vi "Initialize RF Sessions.vi"(0 "RF Subsystem Session Provider in":refnum<class "RF Subsystem Session Provider.lvclass">, 5 "TSM Context":T1, 11 "error in":errorcluster) -> (4 "RF Subsystem Session Provider out":refnum<class "RF Subsystem Session Provider.lvclass">, 15 "error out":errorcluster)   [LabVIEW 2023, in "RFFixtureCharact.RMM.lvlib" / "RF Subsystem Session Provider.lvclass"]
uses:
  RF Subsystem Session Provider.lvclass
  <vilib>/NI_TestStand_SemiconductorModule/NI_TestStand_Semiconductor_Module.lvlibp/PinMap/General/SemiconductorModuleContext.ctl
  Common/RF Subsystem Session Provider/Utilities/Global Data Id Prefix.vi
  <vilib>/NI_TestStand_SemiconductorModule/NI_TestStand_Semiconductor_Module.lvlibp/PinMap/Site and Global Data/SetGlobalData.vi
  RF Subsystem Session Provider.lvclass/RF Subsystem Session Provider.ctl
  <vilib>/NI_TestStand_SemiconductorModule/NI_TestStand_Semiconductor_Module.lvlibp
  Common/RFCalAndFixtureCharact.Common.lvlib
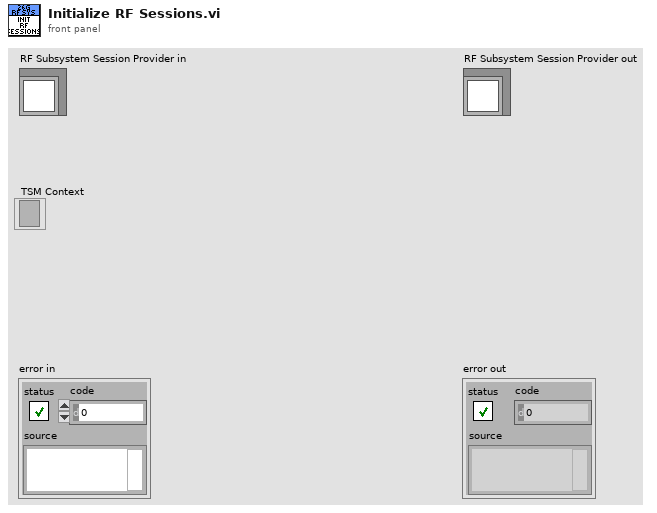
[diagram p1: front panel]
types:
  T1 = typedef "NI_TestStand_Semiconductor_Module.lvlibp/SemiconductorModuleContext.ctl" = refnum<k7>
  T2 = enum16{"OnboardClock", "RefIn", "PXI_Clk", "ClkIn", "RefIn2", "PXI_ClkMaster"}
  T3 = typedef "NI_TestStand_Semiconductor_Module.lvlibp/ModelBasedInstrumentInstanceData.ctl" = cluster{"Instrument Name":string, "Instrument Model":string}
  T4 = typedef "NI_TestStand_Semiconductor_Module.lvlibp/ModelBasedResourcePropertyList.ctl" = cluster{"Instrument Resource":string, "Properties":T5[]}
  T5 = typedef "NI_TestStand_Semiconductor_Module.lvlibp/ModelBasedInstrumentProperty.ctl" = cluster{"Property Name":string, "Property Value":string}
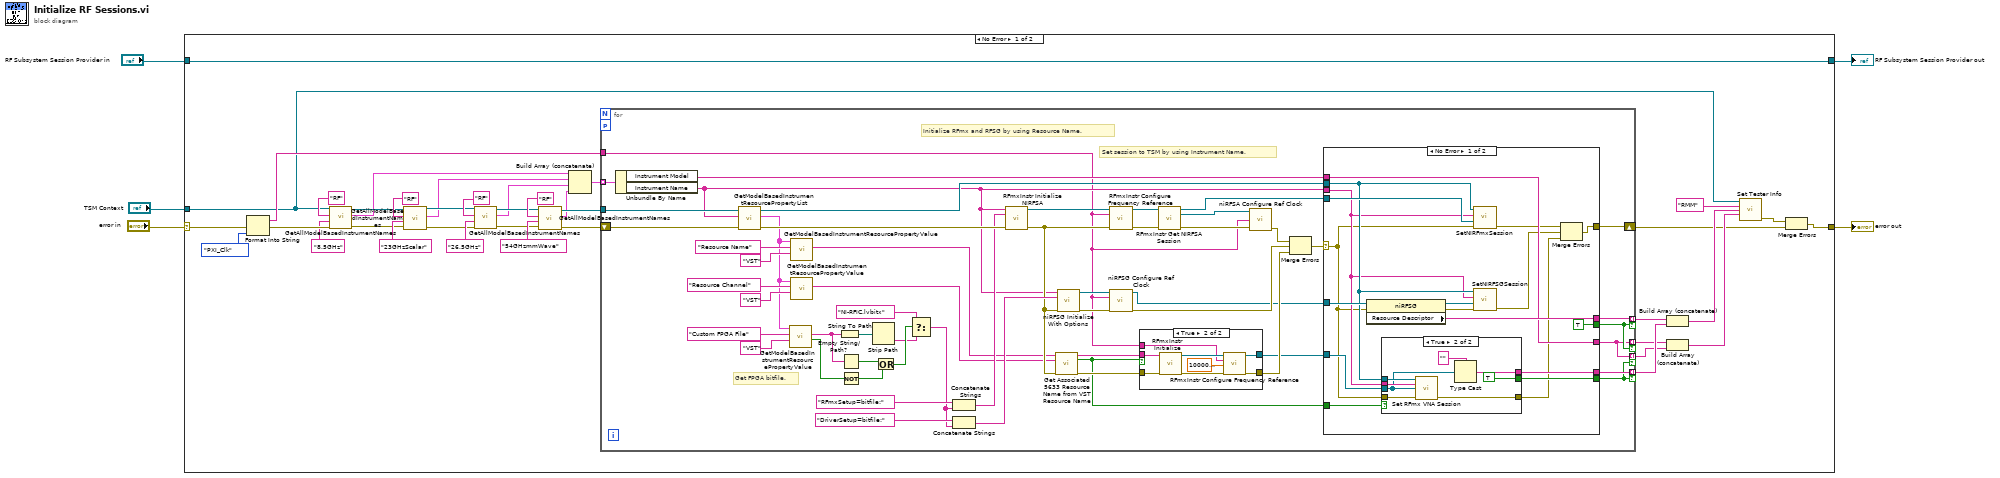
[diagram p0: block diagram]
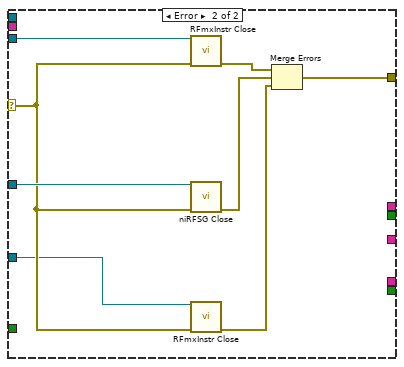
[diagram p3: hidden frame]
diagram:
  n1 = case shown="No Error" "error in" {
    selector: "error in" -> [w39 w142]
    tunnel: [w7 w142] -> w3
    tunnel: "TSM Context" -> [w17 _]
    tunnel: "RF Subsystem Session Provider in" -> [w40 w141]
    tunnel: [w40 w141] -> w1
    frame No Error {
      n2 = Format Into String(error in=w39, T2."PXI_Clk" ("Reference Clock Source In")) -> (resulting string=w37:string, error out=w20:errorcluster)  [unwired: 2 in]
      n3 = call <vilib>:"GetAllModelBasedInstrumentNames.vi"("error in (no error)"=w20, "Subcategory"="8.5GHz", "Category"="RF", "Semiconductor Module Context"=w17) -> ("error out"=w21:errorcluster, "Model-Based Instruments"=w16:T3[], "Semiconductor Module Context Out"=w18:T1)  [unwired: 5 in]
      n4 = call <vilib>:"GetAllModelBasedInstrumentNames.vi"("error in (no error)"=w21, "Subcategory"="23GHzScalar", "Category"="RF", "Semiconductor Module Context"=w18) -> ("error out"=w28:errorcluster, "Model-Based Instruments"=w24:T3[], "Semiconductor Module Context Out"=w25:T1)  [unwired: 5 in]
      n5 = call <vilib>:"GetAllModelBasedInstrumentNames.vi"("error in (no error)"=w28, "Subcategory"="26.5GHz", "Category"="RF", "Semiconductor Module Context"=w25) -> ("error out"=w27:errorcluster, "Model-Based Instruments"=w23:T3[], "Semiconductor Module Context Out"=w26:T1)  [unwired: 5 in]
      n6 = call <vilib>:"GetAllModelBasedInstrumentNames.vi"("error in (no error)"=w27, "Subcategory"="54GHzmmWave", "Category"="RF", "Semiconductor Module Context"=w26) -> ("error out"=w33:errorcluster, "Model-Based Instruments"=w31:T3[], "Semiconductor Module Context Out"=w34:T1)  [unwired: 5 in]
      n7 = Build Array (concatenate)(w16, w24, w23, w31) -> (w32:T3[])
      n8 = for {
        tunnel: w32 -> [w96] mode=indexing
        shift-right: [w49] -> w8
        shift-left: w33 -> [w67]
        workers-P: _ -> [_]
        tunnel: w34 -> [w76]
        tunnel: w37 -> [w43]
        tunnel: [w52] -> w14 mode=indexing if=w46
        tunnel: [w51] -> w15 mode=indexing if=w45
        tunnel: [w44] -> w10 mode=indexing if=w46
        tunnel: [w44] -> w11 mode=indexing if=w45
        # "Set session to TSM by using Instrument Name."
        # "Initialize RFmx and RFSG by using Resource Name."
        # "Get FPGA bitfile."
        n9 = Unbundle By Name(w96) -> ("Instrument Model"=w47:string, "Instrument Name"=w48:string)
        n10 = call <vilib>:"GetModelBasedInstrumentResourcePropertyList.vi"("error in (no error)"=w67, "Instrument Name"=w48, "Semiconductor Module Context"=w76) -> ("error out"=w85:errorcluster, "Model-Based Instrument Resource Property List"=w58:T4[], "Semiconductor Module Context Out"=w54:T1)  [unwired: 6 in]
        n11 = call <vilib>:"GetModelBasedInstrumentResourcePropertyValue.vi"("Resource Name"="VST", "Property Name"="Custom FPGA File", "Model-Based Instrument Resource Property List"=w58) -> ("Is Found"=w90:bool, "Property Value"=w78:string)  [unwired: 6 in, 1 out]
        n12 = call <vilib>:"GetModelBasedInstrumentResourcePropertyValue.vi"("Resource Name"="VST", "Property Name"="Resource Name", "Model-Based Instrument Resource Property List"=w58) -> ("Property Value"=w59:string)  [unwired: 6 in, 2 out]
        n13 = call <vilib>:"GetModelBasedInstrumentResourcePropertyValue.vi"("Resource Name"="VST", "Property Name"="Resource Channel", "Model-Based Instrument Resource Property List"=w58) -> ("Property Value"=w60:string)  [unwired: 6 in, 2 out]
        n14 = String To Path(string=w78) -> (path=w84:path)
        n15 = Empty String/Path?(string/path=w78) -> (empty?=w89:bool)
        n16 = Not(x=w90) -> (.not. x?=w91:bool)
        n17 = Strip Path(path=w84) -> (name=w77:string)  [unwired: 1 out]
        n18 = Or(x=w89, y=w91) -> (x .or. y?=w92:bool)
        n19 = Select(t="NI-RFIC.lvbitx", s=w92, f=w77) -> (s? t:f=w80:string)
        n20 = Concatenate Strings("RFmxSetup=bitfile:" ("format string"), w80) -> (w82:string)
        n21 = Concatenate Strings("DriverSetup=bitfile:" ("option string"), w80) -> (w79:string)
        n22 = call <vilib>:"RFmxInstr Initialize NIRFSA.vi"("Resource Name"=w48, "Option String"=w82, "error in (no error)"=w85) -> ("Instrument Handle Out"=w95:refnum<k21>, "error out"=w65:errorcluster)  [unwired: 10 in, 1 out]
        n23 = call "Get Associated 5633 Resource Name from VST Resource Name.vi"("VST Instrument Name"=w59, "VST Channel"=w60, "error in"=w65) -> ("5633 Resource Name"=w63:string, "Found"=w55:bool, "error out"=w66:errorcluster)  [unwired: 10 in]
        n24 = call <instrlib>:"niRFSG Initialize With Options.vi"("resource name"=w48, "option string"=w79, "error in"=w65) -> ("instrument handle"=w94:refnum<k15>, "error out"=w93:errorcluster)  [unwired: 11 in]
        n25 = call <vilib>:"RFmxInstr Configure Frequency Reference.vi"("Instrument Handle In"=w95, "Frequency Reference Source"=w43, "error in (no error)"=w65) -> ("Instrument Handle Out"=w69:refnum<k21>, "error out"=w68:errorcluster)  [unwired: 11 in]
        n26 = call <instrlib>:"niRFSG Configure Ref Clock.vi"("instrument handle"=w94, "ref clock source"=w43, "error in"=w93) -> ("instrument handle out"=w50:refnum<k15>, "error out"=w70:errorcluster)  [unwired: 11 in]
        n27 = case shown="True" w55 {
          tunnel: w66 -> [w132 w140]
          tunnel: w63 -> [_ w139]
          tunnel: [_ w134] -> w56
          tunnel: [w132 w135] -> w64
          tunnel: w43 -> [_ w133]
          frame False {
          }
          frame True {
            n28 = call <vilib>:"RFmxInstr Initialize.vi"("Resource Name"=w139, "error in (no error)"=w140) -> ("Instrument Handle Out"=w138:refnum<k21>, "error out"=w137:errorcluster)  [unwired: 11 in, 1 out]
            n29 = call <vilib>:"RFmxInstr Configure Frequency Reference.vi"("Instrument Handle In"=w138, "Frequency Reference Source"=w133, "Frequency (Hz)"=100000000.0 ("clock rate"), "error in (no error)"=w137) -> ("Instrument Handle Out"=w134:refnum<k21>, "error out"=w135:errorcluster)  [unwired: 10 in]
          }
        }
        n30 = call <vilib>:"RFmxInstr Get NIRFSA Session.vi"("Instrument Handle In"=w69, "error in (no error)"=w68) -> ("Instrument Handle Out"=w53:refnum<k21>, "NI RFSA Session"=w72:refnum<k15>, "error out"=w73:errorcluster)  [unwired: 11 in]
        n31 = call <instrlib>:"niRFSA Configure Ref Clock.vi"("instrument handle"=w72, "clock source"=w43, "error in"=w73) -> ("error out"=w71:errorcluster)  [unwired: 11 in, 1 out]
        n32 = Merge Errors(w71, w70, w64) -> (w57:errorcluster)
        n33 = case shown="No Error" w57 {
          selector: w57 -> [w101 w126]
          tunnel: [w97 w127] -> w49
          tunnel: w54 -> [w109 _]
          tunnel: w50 -> [w113 w131]
          tunnel: w48 -> [w107 _]
          tunnel: w53 -> [w114 w129]
          tunnel: [w104 _] -> w52
          tunnel: [TRUE _] -> w45
          tunnel: w56 -> [w106 w125]
          tunnel: w55 -> [w108 _]
          tunnel: [w105 _] -> w51
          tunnel: [w103 _] -> w46
          tunnel: w47 -> [w102 _]
          tunnel: [w102 _] -> w44
          frame No Error {
            n34 = property class="niRFSG"(reference=w113, error in=w101) -> (reference out=w112:refnum<k15>, error out=w111:errorcluster, "Resource Descriptor"=w105:string)
            n35 = case shown="True" w108 {
              tunnel: w109 -> [_ w123]
              tunnel: w107 -> [_ w122]
              tunnel: w101 -> [w115 w121]
              tunnel: w106 -> [_ w117]
              tunnel: [w115 w119] -> w98
              tunnel: [_ w118] -> w104
              tunnel: [_ TRUE] -> w103
              frame False {
              }
              frame True {
                n36 = call "Set RFmx VNA Session.vi"("TSM Context"=w123, "VST Instrument Name"=w122, "RFmx VNA Session"=w117, "error in"=w121) -> ("error out"=w119:errorcluster)  [unwired: 11 in]
                n37 = Type Cast(type="", x=w117) -> (*(type *) &x=w118:string)
              }
            }
            n38 = call <vilib>:"SetNIRFmxSession.vi"("error in (no error)"=w101, "NI-RFmx Session"=w114, "Instrument Name"=w107, "Semiconductor Module Context"=w109) -> ("error out"=w100:errorcluster)  [unwired: 6 in, 1 out]
            n39 = call <vilib>:"SetNIRFSGSession.vi"("error in (no error)"=w111, "NI-RFSG Session"=w112, "Instrument Name"=w107, "Semiconductor Module Context"=w109) -> ("error out"=w99:errorcluster)  [unwired: 6 in, 1 out]
            n40 = Merge Errors(w100, w99, w98) -> (w97:errorcluster)
          }
          frame Error {
            n41 = call <vilib>:"RFmxInstr Close.vi"("Instrument Handle In"=w129, "error in (no error)"=w126) -> ("error out"=w130:errorcluster)  [unwired: 13 in]
            n42 = call <instrlib>:"niRFSG Close.vi"("instrument handle"=w131, "error in"=w126) -> ("error out"=w128:errorcluster)  [unwired: 13 in]
            n43 = call <vilib>:"RFmxInstr Close.vi"("Instrument Handle In"=w125, "error in (no error)"=w126) -> ("error out"=w124:errorcluster)  [unwired: 13 in]
            n44 = Merge Errors(w130, w128, w124) -> (w127:errorcluster)
          }
        }
      }
      n45 = Build Array (concatenate)(w15, w14) -> (w12:string[])
      n46 = Build Array (concatenate)(w11, w10) -> (w9:string[])
      n47 = call "Set Tester Info.vi"("TSM Context In"=w17, "Tester Type"="RMM", "Resource Descriptors"=w12, "Instrument Models"=w9) -> ("error out"=w6:errorcluster)  [unwired: 10 in, 1 out]
      n48 = Merge Errors(w6, w8) -> (w7:errorcluster)
    }
    frame Error {
    }
  }
  "error out" <- w3
  "RF Subsystem Session Provider out" <- w1
